vi "Control Panel.vi"(8 "error in (no error)":errorcluster, 11 "Anritsu Optical Power Meter  in":refnum<class "Anritsu Optical Power Meter .lvclass">) -> (0 "error out":errorcluster, 3 "Anritsu Optical Power Meter  out":refnum<class "Anritsu Optical Power Meter .lvclass">)   [LabVIEW 2017, in "Anritsu Optical Power Meter .lvclass"]
doc: "(Dynamic) A user-level application that simulates the physical front panel of the Instrument. Provide the user with buttons to manually control features of the instrument, and provide indicators of its current state."
uses:
  Anritsu Optical Power Meter .lvclass
  Anritsu Power Meter/Public/Display control.ctl
  Anritsu Power Meter/Public/Range control watts and dBm.ctl
  Anritsu Power Meter/Public/Measuring rate control.ctl
  Anritsu Power Meter/Public/Range Status.ctl
  Anritsu Power Meter/Public/Auto Range control.ctl
  Anritsu Power Meter/Public/Averaging control.ctl
  Anritsu Optical Power Meter .lvclass/Anritsu Optical Power Meter .ctl
  Utility Classes/Readable/Readable.lvclass
panel:
  in  "Set Calibration Factor":dbl=-26.67 format="%#5_4g"
  in  "Specify Calibration Factor":bool
  in  "Auto range? 2":bool
  in  "Set Auto Range":T1
  in  "Set Averaging":T2
  out "Averaging":T2
  out "Auto Ranging?":T1
  out "In Range?":T3
  out "Power number":dbl
  out "Power":string
  in  "Set Zero":bool
  in  "Set Unit Range":T4
  in  "Set Measuring Rate":T5
  in  "Specify Range Command":bool
  in  "Set Units":T6
  out "Calibration Factor":dbl
  out "Unit Range":T4
  out "Units":T6
  in  "Query Everything":bool
  in  "Select Measurement Rate":bool
  in  "Averaging?":bool
  in  "Select Unit Display":bool
  in  "Auto range?":bool
  in  "Stop":bool
  in  "Copy actual to set":bool
  in  "Populate fields with member data":bool
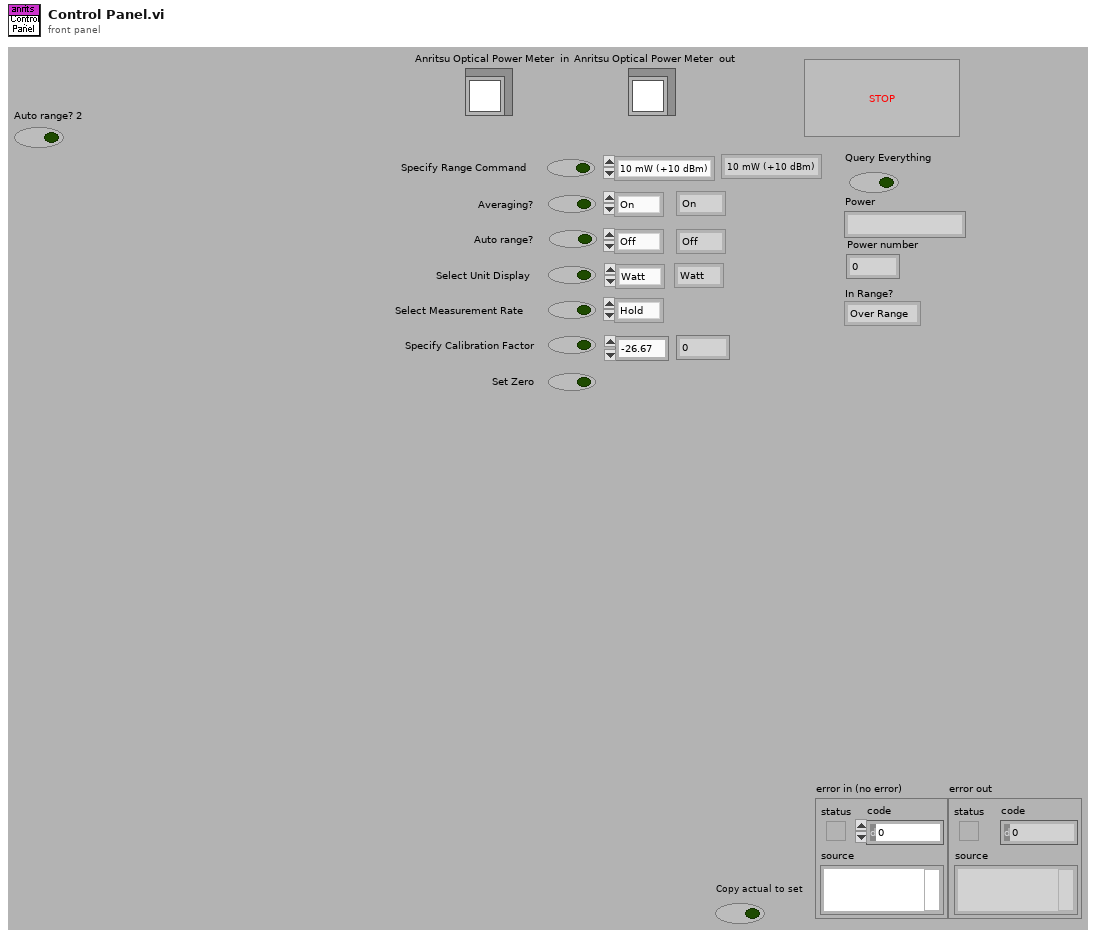
[diagram p1: front panel]
types:
  T1 = typedef "Auto Range control.ctl" = enum16{"Off", "On"}
  T2 = typedef "Averaging control.ctl" = enum16{"On", "Off"}
  T3 = typedef "Range Status.ctl" = enum16{"Over Range", "Under Range", "In Range"}
  T4 = typedef "Range control watts and dBm.ctl" = enum16{"10 mW (+10 dBm)", "1 mW (0 dBm)", "100 uW (-10 dBm)", "10 uW (-20 dBm)", "1 uW (-30 dBm)", "100 nW (-40 dBm)", "10 nW (-50 dBm)", "1 nW (-60 dBm)", "100 pW (-70 dBm)", "10 pW (-80 dBm)"}
  T5 = typedef "Measuring rate control.ctl" = enum16{"Hold", "Free Run", "Exit Trigger"}
  T6 = typedef "Display control.ctl" = enum16{"Watt", "dBm", "dB (REL)"}
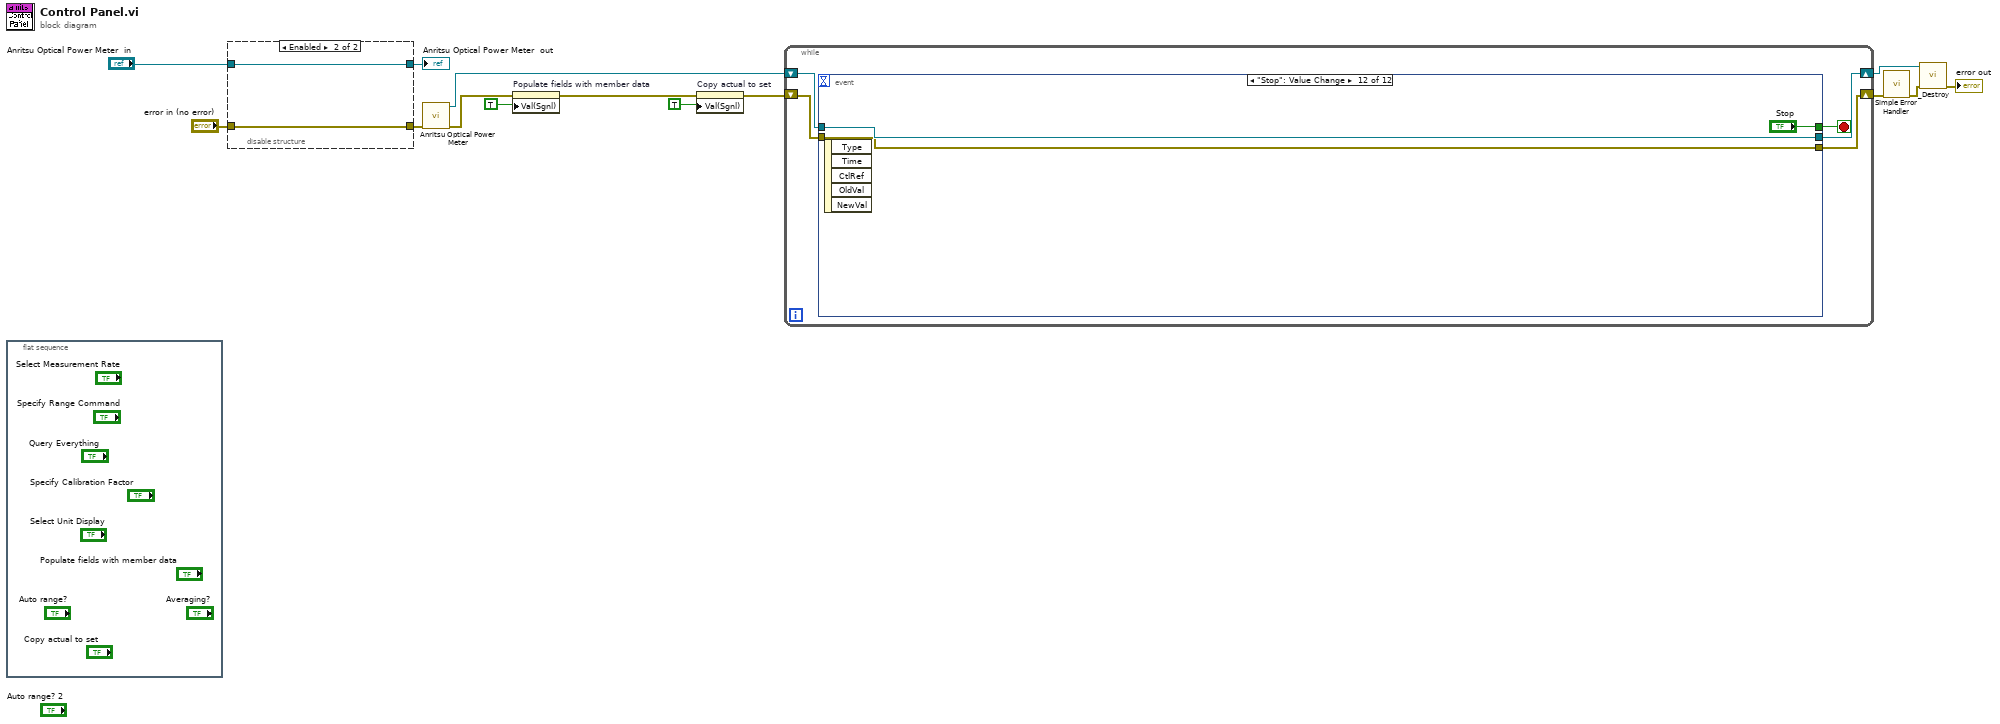
[diagram p0: block diagram]
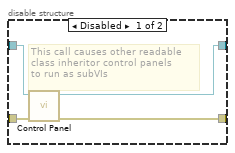
[diagram p2: hidden frame]
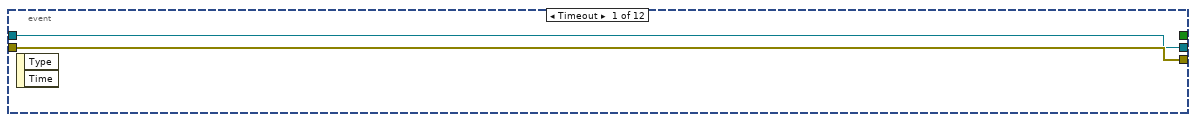
[diagram p3: hidden frame]
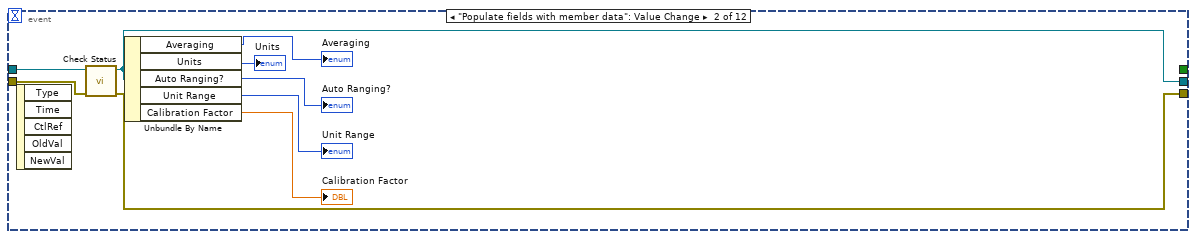
[diagram p4: hidden frame]
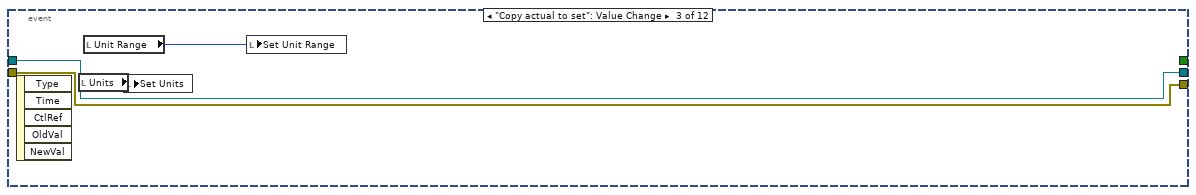
[diagram p5: hidden frame]
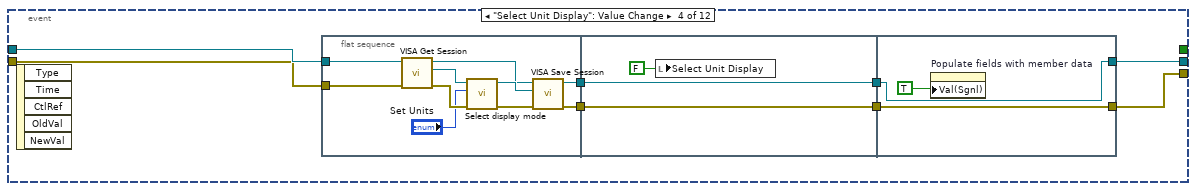
[diagram p6: hidden frame]
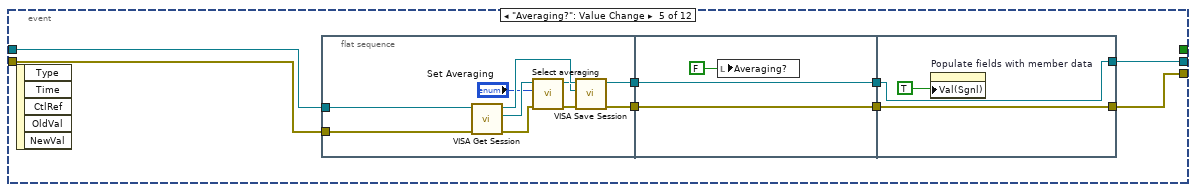
[diagram p7: hidden frame]
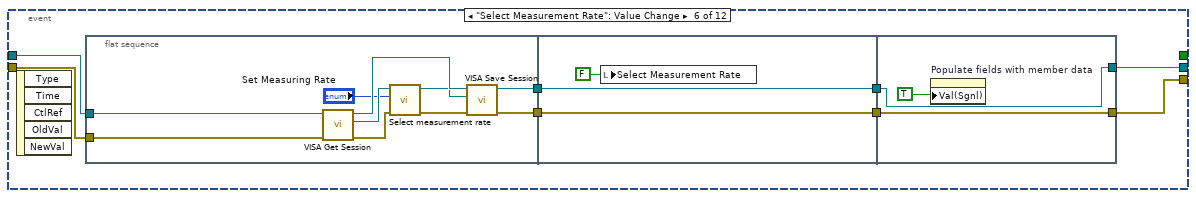
[diagram p8: hidden frame]
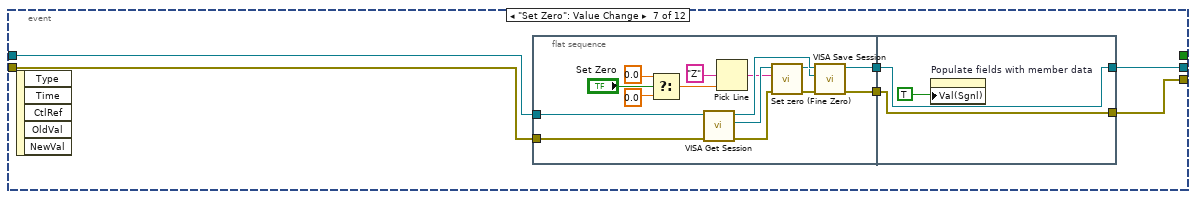
[diagram p9: hidden frame]
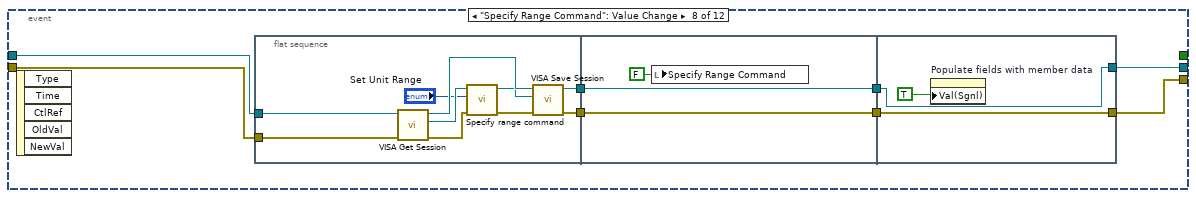
[diagram p10: hidden frame]
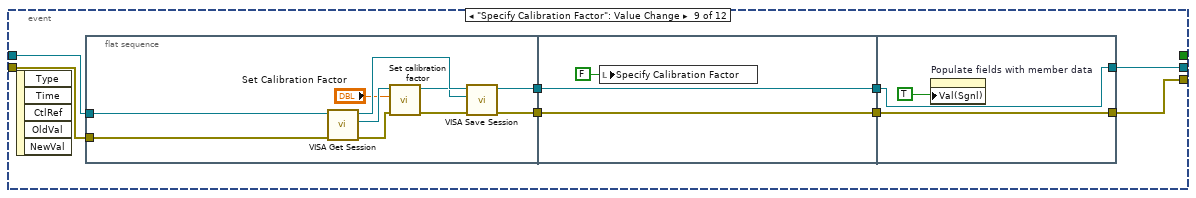
[diagram p11: hidden frame]
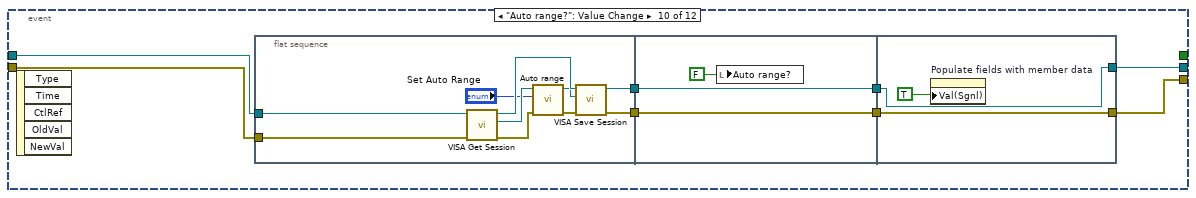
[diagram p12: hidden frame]
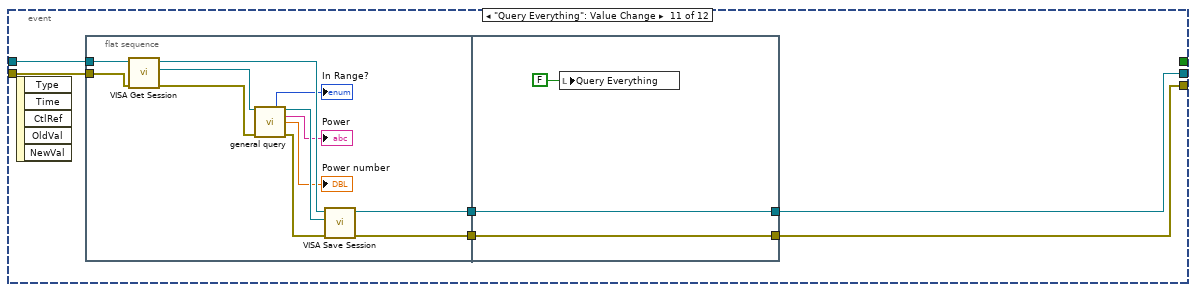
[diagram p13: hidden frame]
diagram:
  n1 = flat-sequence {
    frame #0 {
    }
  }
  n2 = disable-structure shown="Enabled" {
    disable-tunnel: [w18 w20] -> w14
    disable-tunnel: "error in (no error)" -> [w17 w19]
    disable-tunnel: "Anritsu Optical Power Meter  in" -> [w16 w20]
    disable-tunnel: [w15 w19] -> w11
    frame Disabled {
      # "This call causes other readable\nclass inheritor control panels\nto run as subVIs"
      n3 = call-parent "Control Panel.vi"("error in (no error)"=w17, "Instrument in"=w16) -> ("error out"=w15:errorcluster, "Instrument out"=w18:refnum<class "Anritsu Optical Power Meter .lvclass">)  [unwired: 8 in]
    }
    frame Enabled {
    }
  }
  "Anritsu Optical Power Meter  out" <- w14
  n4 = call "Anritsu Optical Power Meter.vi"("error in"=w11) -> ("error out"=w9:errorcluster, "Anritsu Optical Power Meter .lvclass"=w7:refnum<class "Anritsu Optical Power Meter .lvclass">)  [unwired: 9 in]
  n5 = property on="Populate fields with member data" class="Bool (strict)"(error in=w9, "Val(Sgnl)"=TRUE ("Value (Signaling)")) -> (error out=w10:errorcluster)  [unwired: 1 in, 1 out]
  n6 = property on="Copy actual to set" class="Bool (strict)"(error in=w10, "Val(Sgnl)"=TRUE ("Value (Signaling)")) -> (error out=w8:errorcluster)  [unwired: 1 in, 1 out]
  n7 = while {
    shift-right: [w23] -> w4
    shift-left: w7 -> [w24]
    shift-right: [w22] -> w2
    shift-left: w8 -> [w25]
    stop <- w21 stop-if-true
    n8 = event shown="[11] \"Stop\": Value Change" {
      selector: _ -> [_ _ _ _ _ _ _ _ _ _ _ _]
      dyn-events: _ -> [_ _ _ _ _ _ _ _ _ _ _ _]
      timeout: _ -> [_ _ _ _ _ _ _ _ _ _ _ _]
      tunnel: w25 -> [w27 w32 w37 w47 w71 w95 w117 w141 w163 w191 w214 w231]
      tunnel: w24 -> [w26 w33 w38 w48 w72 w96 w118 w142 w164 w192 w213 w232]
      tunnel: [w26 w31 w38 w42 w70 w94 w116 w137 w162 w190 w210 w232] -> w23
      tunnel: [w27 w30 w37 w41 w69 w93 w115 w138 w161 w189 w209 w231] -> w22
      tunnel: [_ _ _ _ _ _ _ _ _ _ _ "Stop"] -> w21
      event Timeout {
        n9 = event-data() -> ()  [unwired: 1 in, 2 out]
      }
      event "Populate fields with member data": Value Change {
        n10 = event-data() -> ()  [unwired: 1 in, 5 out]
        n11 = call-dynamic "Check Status.vi"("error in (no error)"=w32, "Anritsu Optical Power Meter  in"=w33) -> ("error out"=w30:errorcluster, "Anritsu Optical Power Meter  out"=w31:refnum<class "Anritsu Optical Power Meter .lvclass">)  [unwired: 6 in, 2 out]
        n12 = Unbundle By Name(w31) -> ("Averaging"=→"Averaging":T2, "Units"=→"Units":T6, "Auto Ranging?"=→"Auto Ranging?":T1, "Unit Range"=→"Unit Range":T4, "Calibration Factor"=→"Calibration Factor":dbl)
      }
      event "Copy actual to set": Value Change {
        n13 = event-data() -> ()  [unwired: 1 in, 5 out]
        n14 = local read "Units"() -> (w40:T6)
        n15 = local read "Unit Range"() -> (w39:T4)
        n16 = local write "Set Units"(w40) -> ()
        n17 = local write "Set Unit Range"(w39) -> ()
      }
      event "Select Unit Display": Value Change {
        n18 = event-data() -> ()  [unwired: 1 in, 5 out]
        n19 = flat-sequence {
          tunnel: w48 -> [w55]
          tunnel: w47 -> [w56]
          tunnel: [w51] -> w46
          tunnel: [w50] -> w45
          tunnel: w46 -> [w60]
          tunnel: w45 -> [w59]
          tunnel: [w60] -> w44
          tunnel: [w59] -> w43
          tunnel: w44 -> [w63]
          tunnel: w43 -> [w62]
          tunnel: [w63] -> w42
          tunnel: [w62] -> w41
          frame #0 {
            n20 = call-dynamic "VISA Get Session.vi"("error in (no error)"=w56, "Instrument.lvclass in"=w55) -> ("error out"=w58:errorcluster, "VISA Resource Name"=w57:refnum<visa-resource-name>, "Instrument.lvclass out"=w52:refnum<class "Anritsu Optical Power Meter .lvclass">)  [unwired: 7 out]
            n21 = call "Select display mode.vi"("error in (no error)"=w58, "Display"="Set Units", "VISA resource name"=w57) -> ("error out"=w54:errorcluster, "VISA resource name out"=w53:refnum<visa-resource-name>)  [unwired: 7 in]
            n22 = call-dynamic "VISA Save Session.vi"("error in (no error)"=w54, "VISA Resource Name"=w53, "Instrument.lvclass in"=w52) -> ("error out"=w50:errorcluster, "Instrument.lvclass out"=w51:refnum<class "Anritsu Optical Power Meter .lvclass">)  [unwired: 7 out]
          }
          frame #1 {
            n23 = local write "Select Unit Display"(FALSE) -> ()
          }
          frame #2 {
            n24 = property on="Populate fields with member data" class="Bool (strict)"("Val(Sgnl)"=TRUE ("Value (Signaling)")) -> ()  [unwired: 2 in, 2 out]
          }
        }
      }
      event "Averaging?": Value Change {
        n25 = event-data() -> ()  [unwired: 1 in, 5 out]
        n26 = flat-sequence {
          tunnel: w72 -> [w77]
          tunnel: w71 -> [w76]
          tunnel: [w75] -> w68
          tunnel: [w74] -> w66
          tunnel: w68 -> [w85]
          tunnel: [w85] -> w67
          tunnel: w66 -> [w84]
          tunnel: [w84] -> w65
          tunnel: w67 -> [w87]
          tunnel: w65 -> [w86]
          tunnel: [w87] -> w70
          tunnel: [w86] -> w69
          frame #0 {
            n27 = call-dynamic "VISA Get Session.vi"("error in (no error)"=w76, "Instrument.lvclass in"=w77) -> ("error out"=w78:errorcluster, "VISA Resource Name"=w82:refnum<visa-resource-name>, "Instrument.lvclass out"=w81:refnum<class "Anritsu Optical Power Meter .lvclass">)  [unwired: 7 out]
            n28 = call "Select averaging.vi"("error in (no error)"=w78, "Averaging"="Set Averaging", "VISA resource name"=w82) -> ("error out"=w79:errorcluster, "VISA resource name out"=w80:refnum<visa-resource-name>)  [unwired: 7 in]
            n29 = call-dynamic "VISA Save Session.vi"("error in (no error)"=w79, "VISA Resource Name"=w80, "Instrument.lvclass in"=w81) -> ("error out"=w74:errorcluster, "Instrument.lvclass out"=w75:refnum<class "Anritsu Optical Power Meter .lvclass">)  [unwired: 7 out]
          }
          frame #1 {
            n30 = local write "Averaging?"(FALSE) -> ()
          }
          frame #2 {
            n31 = property on="Populate fields with member data" class="Bool (strict)"("Val(Sgnl)"=TRUE ("Value (Signaling)")) -> ()  [unwired: 2 in, 2 out]
          }
        }
      }
      event "Select Measurement Rate": Value Change {
        n32 = event-data() -> ()  [unwired: 1 in, 5 out]
        n33 = flat-sequence {
          tunnel: w96 -> [w101]
          tunnel: w95 -> [w100]
          tunnel: [w98] -> w92
          tunnel: [w97] -> w90
          tunnel: w92 -> [w109]
          tunnel: [w109] -> w91
          tunnel: w90 -> [w108]
          tunnel: [w108] -> w89
          tunnel: w91 -> [w111]
          tunnel: w89 -> [w110]
          tunnel: [w111] -> w94
          tunnel: [w110] -> w93
          frame #0 {
            n34 = call-dynamic "VISA Get Session.vi"("error in (no error)"=w100, "Instrument.lvclass in"=w101) -> ("error out"=w102:errorcluster, "VISA Resource Name"=w105:refnum<visa-resource-name>, "Instrument.lvclass out"=w106:refnum<class "Anritsu Optical Power Meter .lvclass">)  [unwired: 7 out]
            n35 = call "Select measurement rate.vi"("error in (no error)"=w102, "Rate"="Set Measuring Rate", "VISA resource name"=w105) -> ("error out"=w103:errorcluster, "VISA resource name out"=w104:refnum<visa-resource-name>)  [unwired: 7 in]
            n36 = call-dynamic "VISA Save Session.vi"("error in (no error)"=w103, "VISA Resource Name"=w104, "Instrument.lvclass in"=w106) -> ("error out"=w97:errorcluster, "Instrument.lvclass out"=w98:refnum<class "Anritsu Optical Power Meter .lvclass">)  [unwired: 7 out]
          }
          frame #1 {
            n37 = local write "Select Measurement Rate"(FALSE) -> ()
          }
          frame #2 {
            n38 = property on="Populate fields with member data" class="Bool (strict)"("Val(Sgnl)"=TRUE ("Value (Signaling)")) -> ()  [unwired: 2 in, 2 out]
          }
        }
      }
      event "Set Zero": Value Change {
        n39 = event-data() -> ()  [unwired: 1 in, 5 out]
        n40 = flat-sequence {
          tunnel: w117 -> [w128]
          tunnel: w118 -> [w127]
          tunnel: [w126] -> w114
          tunnel: [w125] -> w113
          tunnel: w114 -> [w135]
          tunnel: w113 -> [w134]
          tunnel: [w135] -> w116
          tunnel: [w134] -> w115
          frame #0 {
            n41 = Select(t=0.0, s="Set Zero", f=0.0) -> (s? t:f=w122:dbl)
            n42 = call-dynamic "VISA Get Session.vi"("error in (no error)"=w128, "Instrument.lvclass in"=w127) -> ("error out"=w129:errorcluster, "VISA Resource Name"=w132:refnum<visa-resource-name>, "Instrument.lvclass out"=w133:refnum<class "Anritsu Optical Power Meter .lvclass">)  [unwired: 7 out]
            n43 = Pick Line(multi-line string="Z", line index=w122) -> (output string=w120:string)  [unwired: 1 in]
            n44 = call "Set zero (Fine Zero).vi"("error in (no error)"=w129, "Code"=w120, "VISA resource name"=w132) -> ("error out"=w130:errorcluster, "VISA resource name out"=w131:refnum<visa-resource-name>)  [unwired: 7 in]
            n45 = call-dynamic "VISA Save Session.vi"("error in (no error)"=w130, "VISA Resource Name"=w131, "Instrument.lvclass in"=w133) -> ("error out"=w125:errorcluster, "Instrument.lvclass out"=w126:refnum<class "Anritsu Optical Power Meter .lvclass">)  [unwired: 7 out]
          }
          frame #1 {
            n46 = property on="Populate fields with member data" class="Bool (strict)"("Val(Sgnl)"=TRUE ("Value (Signaling)")) -> ()  [unwired: 2 in, 2 out]
          }
        }
      }
      event "Specify Range Command": Value Change {
        n47 = event-data() -> ()  [unwired: 1 in, 5 out]
        n48 = flat-sequence {
          tunnel: [w154] -> w144
          tunnel: [w153] -> w143
          tunnel: w142 -> [w152]
          tunnel: w141 -> [w151]
          tunnel: w144 -> [w156]
          tunnel: w143 -> [w155]
          tunnel: [w156] -> w140
          tunnel: [w155] -> w139
          tunnel: w140 -> [w159]
          tunnel: w139 -> [w158]
          tunnel: [w159] -> w137
          tunnel: [w158] -> w138
          frame #0 {
            n49 = call-dynamic "VISA Get Session.vi"("error in (no error)"=w151, "Instrument.lvclass in"=w152) -> ("error out"=w146:errorcluster, "VISA Resource Name"=w149:refnum<visa-resource-name>, "Instrument.lvclass out"=w150:refnum<class "Anritsu Optical Power Meter .lvclass">)  [unwired: 7 out]
            n50 = call "Specify range command.vi"("error in (no error)"=w146, "Range"="Set Unit Range", "VISA resource name"=w149) -> ("error out"=w147:errorcluster, "VISA resource name out"=w148:refnum<visa-resource-name>)  [unwired: 7 in]
            n51 = call-dynamic "VISA Save Session.vi"("error in (no error)"=w147, "VISA Resource Name"=w148, "Instrument.lvclass in"=w150) -> ("error out"=w153:errorcluster, "Instrument.lvclass out"=w154:refnum<class "Anritsu Optical Power Meter .lvclass">)  [unwired: 7 out]
          }
          frame #1 {
            n52 = local write "Specify Range Command"(FALSE) -> ()
          }
          frame #2 {
            n53 = property on="Populate fields with member data" class="Bool (strict)"("Val(Sgnl)"=TRUE ("Value (Signaling)")) -> ()  [unwired: 2 in, 2 out]
          }
        }
      }
      event "Specify Calibration Factor": Value Change {
        n54 = event-data() -> ()  [unwired: 1 in, 5 out]
        n55 = flat-sequence {
          tunnel: [w178] -> w168
          tunnel: [w177] -> w167
          tunnel: w164 -> [w171]
          tunnel: w163 -> [w170]
          tunnel: w168 -> [w181]
          tunnel: [w181] -> w166
          tunnel: w167 -> [w180]
          tunnel: [w180] -> w165
          tunnel: w166 -> [w184]
          tunnel: w165 -> [w183]
          tunnel: [w184] -> w162
          tunnel: [w183] -> w161
          frame #0 {
            n56 = call-dynamic "VISA Get Session.vi"("error in (no error)"=w170, "Instrument.lvclass in"=w171) -> ("error out"=w172:errorcluster, "VISA Resource Name"=w175:refnum<visa-resource-name>, "Instrument.lvclass out"=w176:refnum<class "Anritsu Optical Power Meter .lvclass">)  [unwired: 7 out]
            n57 = call "Set calibration factor.vi"("error in (no error)"=w172, "Calibration Factor"="Set Calibration Factor", "VISA resource name"=w175) -> ("error out"=w173:errorcluster, "VISA resource name out"=w174:refnum<visa-resource-name>)  [unwired: 7 in]
            n58 = call-dynamic "VISA Save Session.vi"("error in (no error)"=w173, "VISA Resource Name"=w174, "Instrument.lvclass in"=w176) -> ("error out"=w177:errorcluster, "Instrument.lvclass out"=w178:refnum<class "Anritsu Optical Power Meter .lvclass">)  [unwired: 7 out]
          }
          frame #1 {
            n59 = local write "Specify Calibration Factor"(FALSE) -> ()
          }
          frame #2 {
            n60 = property on="Populate fields with member data" class="Bool (strict)"("Val(Sgnl)"=TRUE ("Value (Signaling)")) -> ()  [unwired: 2 in, 2 out]
          }
        }
      }
      event "Auto range?": Value Change {
        n61 = event-data() -> ()  [unwired: 1 in, 5 out]
        n62 = flat-sequence {
          tunnel: [w202] -> w188
          tunnel: [w201] -> w186
          tunnel: w192 -> [w198]
          tunnel: w191 -> [w199]
          tunnel: w188 -> [w205]
          tunnel: [w205] -> w187
          tunnel: w186 -> [w204]
          tunnel: [w204] -> w185
          tunnel: w187 -> [w208]
          tunnel: w185 -> [w207]
          tunnel: [w208] -> w190
          tunnel: [w207] -> w189
          frame #0 {
            n63 = call-dynamic "VISA Get Session.vi"("error in (no error)"=w199, "Instrument.lvclass in"=w198) -> ("error out"=w196:errorcluster, "VISA Resource Name"=w197:refnum<visa-resource-name>, "Instrument.lvclass out"=w200:refnum<class "Anritsu Optical Power Meter .lvclass">)  [unwired: 7 out]
            n64 = call "Auto range.vi"("error in (no error)"=w196, "Auto Ranging?"="Set Auto Range", "VISA resource name"=w197) -> ("error out"=w195:errorcluster, "VISA resource name out"=w194:refnum<visa-resource-name>)  [unwired: 7 in]
            n65 = call-dynamic "VISA Save Session.vi"("error in (no error)"=w195, "VISA Resource Name"=w194, "Instrument.lvclass in"=w200) -> ("error out"=w201:errorcluster, "Instrument.lvclass out"=w202:refnum<class "Anritsu Optical Power Meter .lvclass">)  [unwired: 7 out]
          }
          frame #1 {
            n66 = local write "Auto range?"(FALSE) -> ()
          }
          frame #2 {
            n67 = property on="Populate fields with member data" class="Bool (strict)"("Val(Sgnl)"=TRUE ("Value (Signaling)")) -> ()  [unwired: 2 in, 2 out]
          }
        }
      }
      event "Query Everything": Value Change {
        n68 = event-data() -> ()  [unwired: 1 in, 5 out]
        n69 = flat-sequence {
          tunnel: w214 -> [w223]
          tunnel: w213 -> [w222]
          tunnel: [w219] -> w212
          tunnel: [w218] -> w211
          tunnel: w212 -> [w227]
          tunnel: w211 -> [w228]
          tunnel: [w228] -> w210
          tunnel: [w227] -> w209
          frame #0 {
            n70 = call-dynamic "VISA Get Session.vi"("error in (no error)"=w223, "Instrument.lvclass in"=w222) -> ("error out"=w224:errorcluster, "VISA Resource Name"=w225:refnum<visa-resource-name>, "Instrument.lvclass out"=w226:refnum<class "Anritsu Optical Power Meter .lvclass">)  [unwired: 7 out]
            n71 = call "general query.vi"("VISA resource name"=w225, "error in (no error)"=w224) -> ("In Range?"=→"In Range?":T3, "VISA resource name out"=w221:refnum<visa-resource-name>, "Power"=→"Power":string, "Power num"=→"Power number":dbl, "error out"=w220:errorcluster)  [unwired: 5 in, 4 out]
            n72 = call-dynamic "VISA Save Session.vi"("error in (no error)"=w220, "VISA Resource Name"=w221, "Instrument.lvclass in"=w226) -> ("error out"=w219:errorcluster, "Instrument.lvclass out"=w218:refnum<class "Anritsu Optical Power Meter .lvclass">)  [unwired: 7 out]
          }
          frame #1 {
            n73 = local write "Query Everything"(FALSE ("Value (Signaling)")) -> ()
          }
        }
      }
      event "Stop": Value Change {
        n74 = event-data() -> ()  [unwired: 1 in, 5 out]
      }
    }
  }
  n75 = call <vilib>:"Simple Error Handler.vi"("error in (no error)"=w2) -> ("error out"=w3:errorcluster)  [unwired: 1 in, 7 out]
  n76 = call-dynamic "_Destroy.vi"("error in (no error)"=w3, "Instrument in"=w4) -> ("error out"=→"error out":errorcluster)  [unwired: 9 out]
